vi "Autonomous Independent.vi"() -> ()   [LabVIEW 2020]
doc: "This VI is called when autonomous begins, and will automatically be terminated when autonomous ends. You can carry out timed or sensor driven robot movement independently without needing to return to the caller."
uses:
  <vilib>/Rock Robotics/WPI/Utilities/WPI_GetSetVariantRefNum.vi
  Globals/FilePath_Globals.vi
panel:
  out "Name of Play":string
  out "DS Message":string
  out "Done":bool
  # "Be sure to right-click and choose Data Operations>>Make Current Value default if you want to save the array values with the VI"
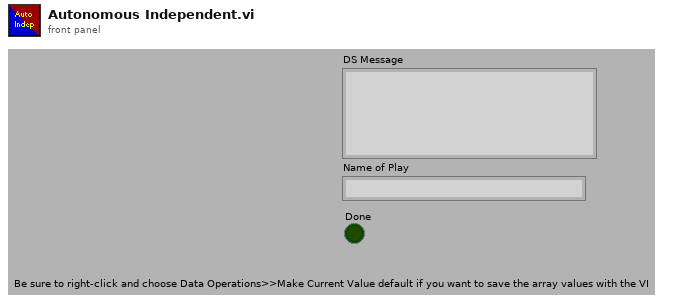
[diagram p1: front panel]
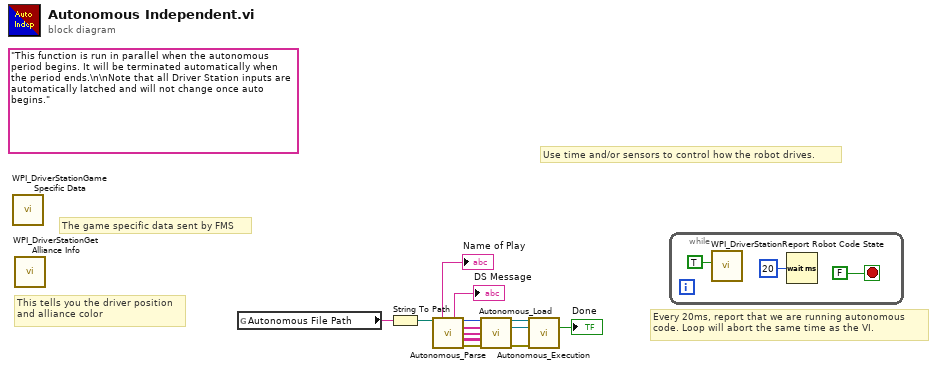
[diagram p0: block diagram]
diagram:
  (unwired) "This function is run in parallel when the autonomous period begins. It will be terminated automatically when the period ends.\n\nNote that all Driver Station inputs are automatically latched and will not change once auto begins."
  # "The game specific data sent by FMS"
  # "Every 20ms, report that we are running autonomous\ncode. Loop will abort the same time as the VI."
  # "Use time and/or sensors to control how the robot drives."
  # "This tells you the driver position\nand alliance color"
  n1 = call <vilib>:"WPI_DriverStationGame Specific Data.vi"() -> ()  [unwired: 11 in, 1 out]
  n2 = call <vilib>:"WPI_DriverStationGet Alliance Info.vi"() -> ()  [unwired: 12 out]
  n3 = global read "FilePath_Globals.vi" "Autonomous File Path"() -> (w2:string)
  n4 = String To Path(string=w2) -> (path=w1:path)
  n5 = call "Autonomous_Parse.vi"("File Path"=w1) -> ("Name of Play"=→"Name of Play":string, "DS Message"=→"DS Message":string, "Number of Commands"=w13:i32, "Subsystems"=w12:string[], "Commands"=w11:string[], "Inputs"=w10:string[][], "errror out"=w9:errorcluster)  [unwired: 8 in]
  n6 = call "Autonomous_Load.vi"("Number of Commands"=w13, "Subsystems"=w12, "Commands"=w11, "Inputs"=w10, "error in"=w9) -> ("Queue_Key"=w6:refnum<queue>, "Autonomous_Queue"=w7:refnum<queue>, "errror out"=w8:errorcluster)  [unwired: 8 in]
  n7 = call "Autonomous_Execution.vi"("Queue Key"=w6, "Autonomous_Queue"=w7, "error in"=w8) -> ("Done"=→"Done":bool)  [unwired: 12 in]
  n8 = while {
    stop <- FALSE stop-if-true
    n9 = call <vilib>:"WPI_DriverStationReport Robot Code State.vi"("Autonomous"=TRUE) -> ()  [unwired: 10 in, 1 out]
    n10 = Wait (ms)(milliseconds to wait=u32 20) -> ()  [unwired: 1 out]
  }
